vi "Configure Slider_Steering.vi"(8 "error in (no error)":errorcluster, 9 "NIVS.System Definition Root":refnum<k24>, 10 "VI Reference":refnum<vi>, 11 "Slide Parameters In":T1) -> (0 "error out":errorcluster, 3 "Slide Parameters Out":T1)   [LabVIEW 2013]
doc: "Use this template to create a dialog box with event handling."
uses:
  NationalInstruments.VeriStand.SystemStorage
  Support/Slide Parameters.ctl
  Support/PWM Object Parameters.ctl
  <vilib>/NI Veristand/UI Controls/Single Node Browser/NI_VS UI Single Node Browser.lvlib
  NationalInstruments.VeriStand.SystemStorageUI
panel:
  in  "Make Current Values Default":bool
  in  "Min Rail":dbl=0.1 min=0.0 max=1.0 step=0.0001
  in  "Max Rail":dbl=0.9 min=0.0 max=1.0 step=0.0001
  in  "BG color":u32(colorbox)=1245174
  in  "RIO?":bool caption="Hardware type"
  in  "Control Label":string
  out "PWM Config Tab":enum32{"DAQ", "RIO"}(tab)=enum."RIO"
  in  "OK":bool
  in  "Cancel":bool
  in  "Selected Channel":refnum<k24>(container)
  # "PWM Duty Cycle"
  # "LEFT"
  # "RIGHT"
  # "DAQ\nPWM\nRatio"
  # "FPGA\nPWM\n%"
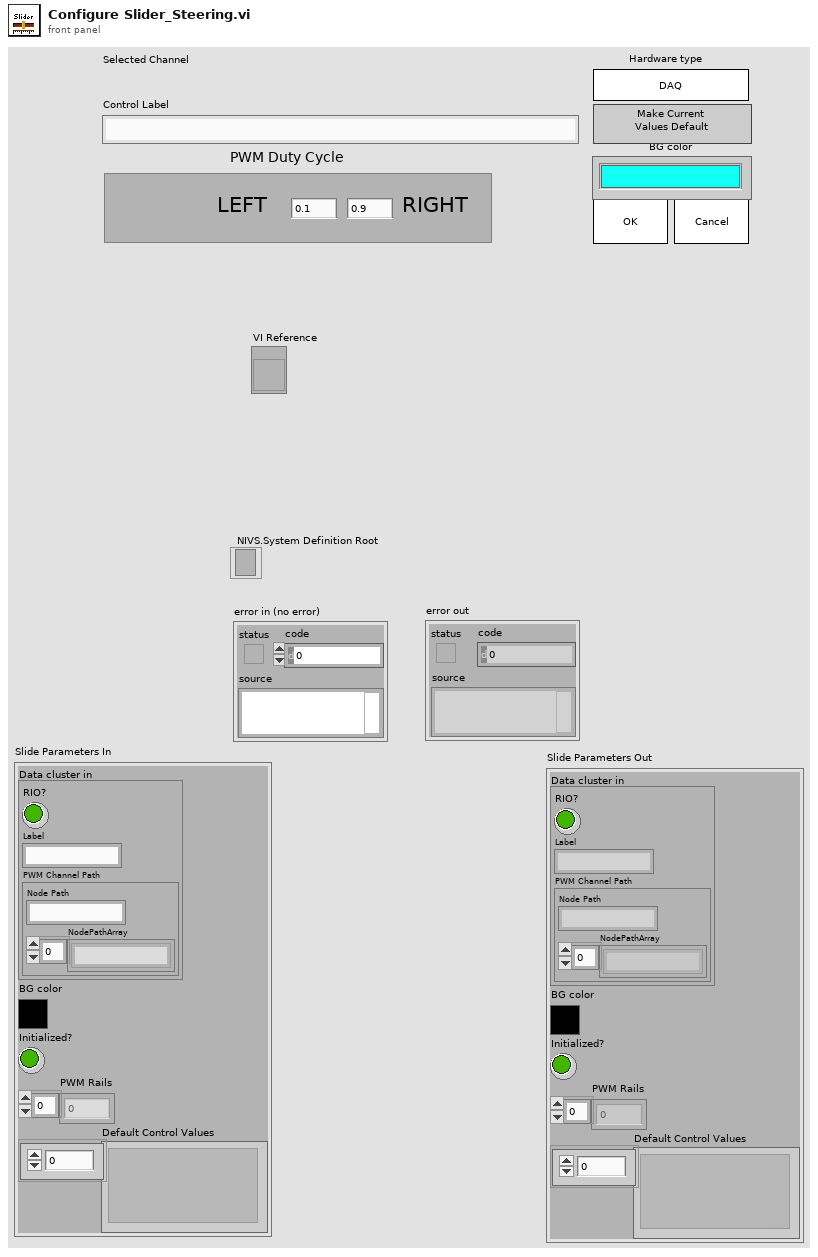
[diagram p1: front panel]
types:
  T1 = typedef "Slide Parameters.ctl" = cluster{"Data cluster in":T2, "BG color":u32, "Initialized?":bool, "PWM Rails":dbl[], "Default Control Values":variant[]}
  T2 = typedef "PWM Object Parameters.ctl" = cluster{"RIO?":bool, "Label":string, "PWM Channel Path":cluster{"NodePathArray":string[], "Node Path":string}}
  T3 = typedef "NI_VS UI Single Node Browser.lvlib/Callback Type.ctl" = cluster{"Net Callbacks":refnum<k27>[], "Event":refnum<user-event>}
  T4 = typedef "NI_VS UI Single Node Browser.lvlib/Node Ref.ctl" = refnum<k24>
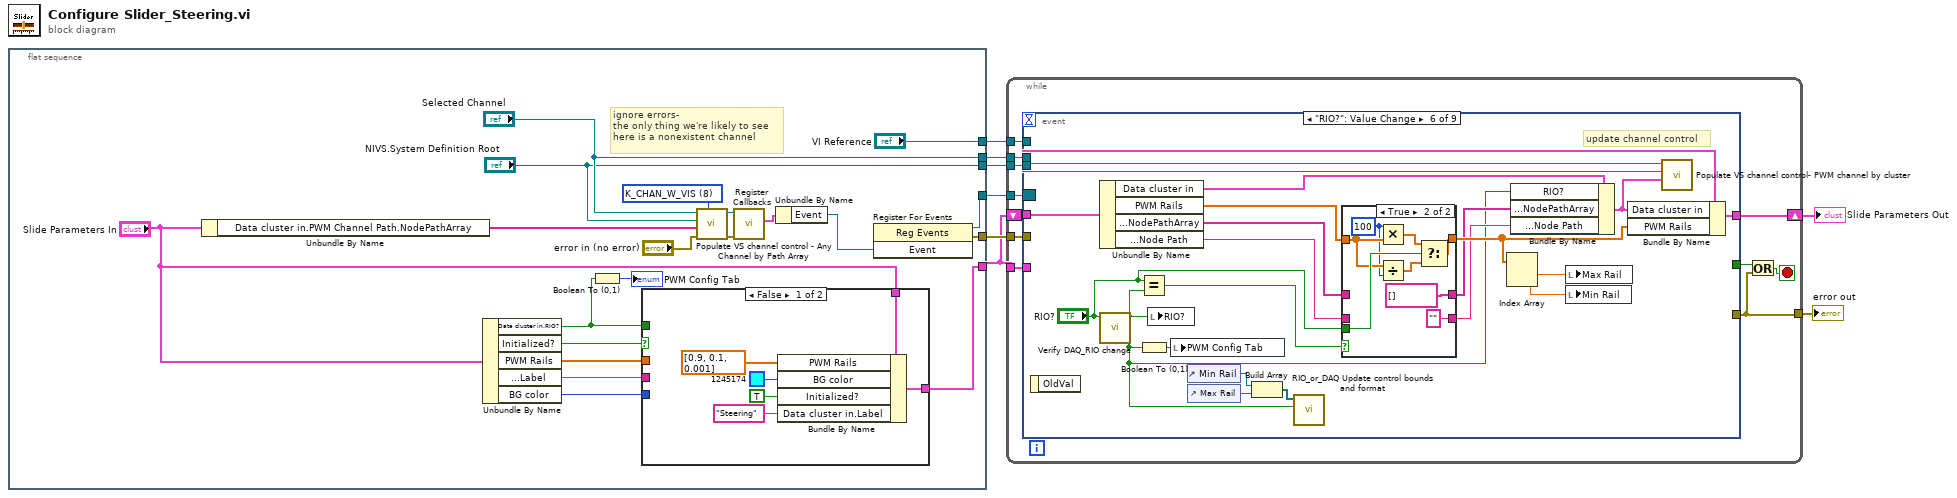
[diagram p0: block diagram]
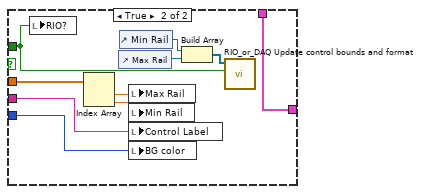
[diagram p2: hidden frame]
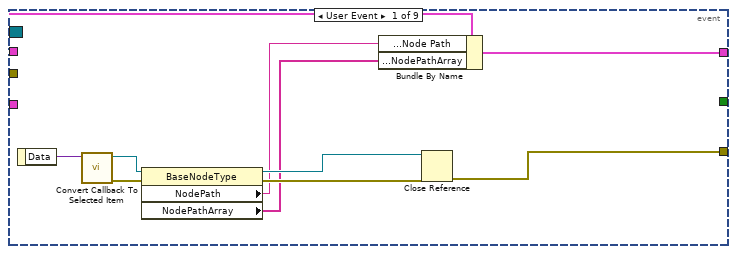
[diagram p3: hidden frame]
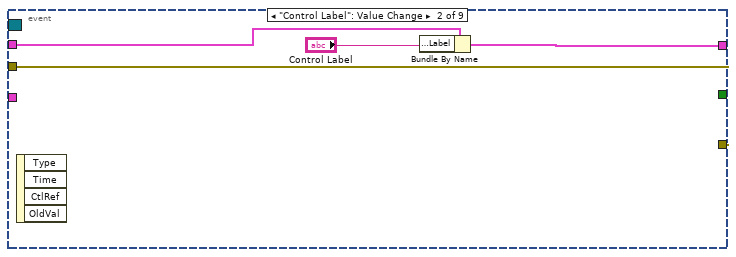
[diagram p4: hidden frame]
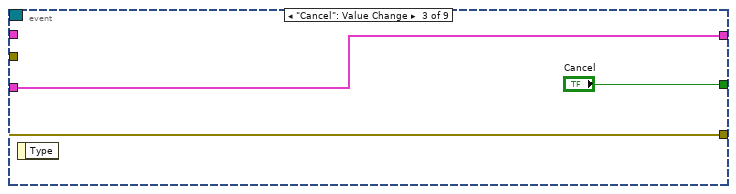
[diagram p5: hidden frame]
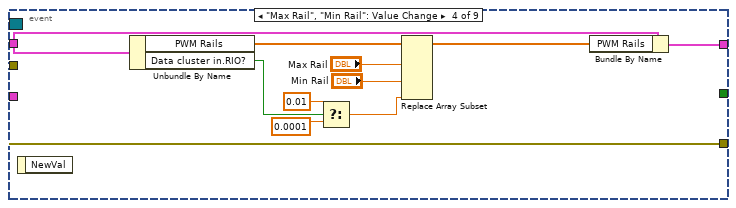
[diagram p6: hidden frame]
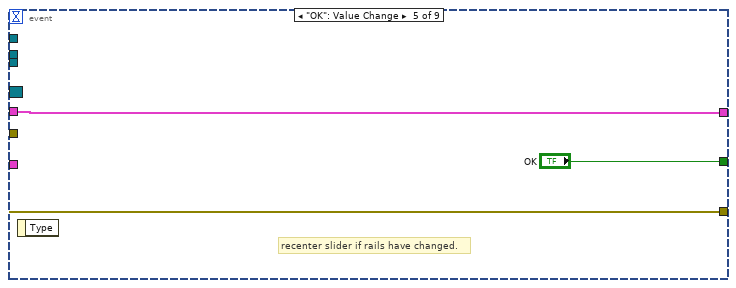
[diagram p7: hidden frame]
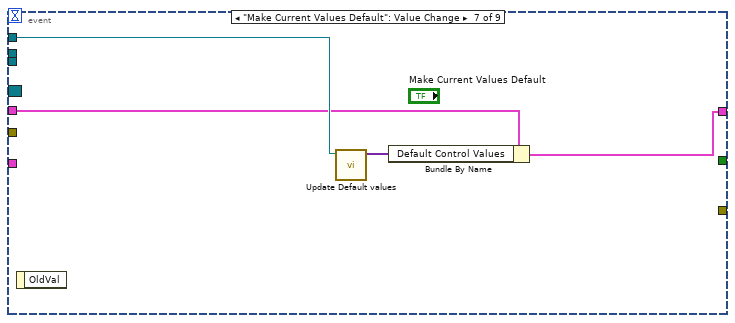
[diagram p9: hidden frame]
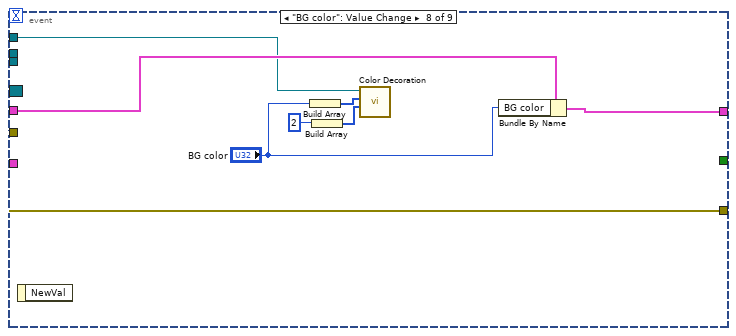
[diagram p10: hidden frame]
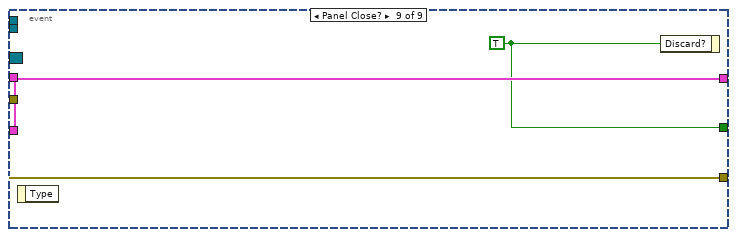
[diagram p11: hidden frame]
diagram:
  n1 = flat-sequence {
    tunnel: ["Selected Channel"] -> w7
    tunnel: ["NIVS.System Definition Root"] -> w6
    tunnel: [w13] -> w5
    tunnel: [w19] -> w4
    tunnel: ["VI Reference"] -> w3
    tunnel: [w12] -> w2
    frame #0 {
      w26 = u8 8 items=["K_CHAN_R", "K_CHAN_W", "K_CHAN_RW", "K_CHAN_VOLT", "K_CHAN_FAULT", "K_ALL", "K_CUSTOM", "K_CHAN_R_VIS", "K_CHAN_W_VIS", "K_CHAN_RW_VIS", "K_CHAN_VOLT_VIS", "K_CHAN_FAULT_VIS"] ("DisplayFilter")
      # "ignore errors-\nthe only thing we're likely to see\nhere is a nonexistent channel"
      n2 = Unbundle By Name("Slide Parameters In") -> ("Data cluster in.PWM Channel Path.NodePathArray"=w9:string[])
      n3 = Unbundle By Name("Slide Parameters In") -> ("Data cluster in.RIO?"=w10:bool, "Initialized?"=w20:bool, "PWM Rails"=w23:dbl[], "Data cluster in.Label"=w22:string, "BG color"=w21:u32)
      n4 = Boolean To (0,1)(Boolean=w10) -> (0, 1=→"PWM Config Tab":i16)
      n5 = case shown="False" w20 {
        tunnel: w23 -> [_ w43]
        tunnel: w22 -> [_ w42]
        tunnel: w21 -> [_ w41]
        tunnel: "Slide Parameters In" -> [w34 w40]
        tunnel: [w33 w40] -> w19
        tunnel: w10 -> [_ w37]
        frame False {
          n6 = Bundle By Name(cluster=w34, "PWM Rails"=dbl[] [0.9, 0.1, 0.001] ("RIO PWM Settings"), "BG color"=u32 1245174, "Initialized?"=TRUE ("New?"), "Data cluster in.Label"="Steering" ("Label")) -> (w33:T1)
        }
        frame True {
          n7 = local write "RIO?"(w37) -> ()
          n8 = Index Array(array=w43) -> (element #1=w44:dbl, element #2=w39:dbl)  [unwired: 2 in]
          n9 = control-ref of="Max Rail"() -> (w35:refnum<vi>)
          n10 = control-ref of="Min Rail"() -> (w36:refnum<vi>)
          n11 = local write "Max Rail"(w44) -> ()
          n12 = local write "Min Rail"(w39) -> ()
          n13 = local write "Control Label"(w42) -> ()
          n14 = local write "BG color"(w41) -> ()
          n15 = Build Array(w36, w35) -> (w38:refnum<vi>[])
          n16 = call "RIO_or_DAQ Update control bounds and format.vi"("RIO? in"=w37, "Control References in"=w38) -> ()  [unwired: 10 in]
        }
      }
      n17 = call "Populate VS channel control - Any Channel by Path Array.vi"("DisplayFilter"=w26, "error in (no error)"="error in (no error)", "Path Array In"=w9, "NIVS.System Definition Root"="NIVS.System Definition Root", ".NET Refnum in"="Selected Channel") -> ("error out"=w14:errorcluster, ".NET Refnum out"=w15:refnum<k24>)  [unwired: 5 in]
      n18 = call <vilib>:"Register Callbacks.vi"("error in (no error)"=w14, "Single Node Browser"=w15) -> ("Callbacks"=w17:T3)  [unwired: 7 in, 2 out]
      n19 = Unbundle By Name(w17) -> ("Event"=w16:refnum<user-event>)
      n20 = register-events(w16) -> (reference out=w12:refnum<event-registration>, error out=w13:errorcluster)  [unwired: 2 in]
    }
  }
  n21 = while {
    tunnel: [w45] -> w8
    shift-right: [w52] -> w1
    shift-left: w4 -> [w54]
    tunnel: w4 -> [w53]
    tunnel: w7 -> [w50]
    tunnel: w6 -> [w49]
    tunnel: w5 -> [w48]
    tunnel: w3 -> [w47]
    tunnel: w2 -> [w46]
    stop <- w51 stop-if-true
    n22 = event shown="[5] \"RIO?\": Value Change" {
      selector: w46 -> [_ _ _ _ _ _ _ _ _]
      dyn-events: _ -> [_ _ _ _ _ _ _ _ _]
      timeout: _ -> [_ _ _ _ _ _ _ _ _]
      tunnel: [_ _ "Cancel" _ "OK" _ _ _ w132] -> w55
      tunnel: [w57 w66 w70 w83 w85 _ _ w128 w131] -> w45
      tunnel: w54 -> [w58 w68 _ w81 w84 w104 w120 w129 _]
      tunnel: w53 -> [_ _ w71 _ _ _ _ _ w133]
      tunnel: [w56 w69 w71 w82 w84 w105 w119 w130 w133] -> w52
      tunnel: w50 -> [_ _ _ _ _ w107 _ _ _]
      tunnel: w49 -> [_ _ _ _ _ w106 _ _ _]
      tunnel: w48 -> [_ w66 w70 w83 w85 _ _ w128 w131]
      tunnel: w47 -> [_ _ _ _ _ _ w121 w125 _]
      event User Event {
        n23 = event-data() -> ("Data"=w59:variant)  [unwired: 1 in]
        n24 = call <vilib>:"Convert Callback To Selected Item.vi"("Data"=w59) -> ("error out"=w62:errorcluster, "Selected Item"=w65:T4)  [unwired: 9 in]
        n25 = property class="BaseNodeType"(reference=w65, error in=w62) -> (reference out=w64:T4, error out=w63:errorcluster, "NodePath"=w61:string, "NodePathArray"=w60:string[])
        n26 = Bundle By Name(cluster=w58, "Data cluster in.PWM Channel Path.Node Path"=w61, "Data cluster in.PWM Channel Path.NodePathArray"=w60) -> (w56:T1)
        n27 = Close Reference(reference=w64, error in (no error)=w63) -> (error out=w57:errorcluster)
      }
      event "Control Label": Value Change {
        n28 = event-data() -> ()  [unwired: 1 in, 4 out]
        n29 = Bundle By Name(cluster=w68, "Data cluster in.Label"="Control Label") -> (w69:T1)
      }
      event "Cancel": Value Change {
        n30 = event-data() -> ()  [unwired: 1 in, 1 out]
      }
      event "Max Rail", "Min Rail": Value Change {
        n31 = event-data() -> ()  [unwired: 1 in, 1 out]
        n32 = Unbundle By Name(w81) -> ("PWM Rails"=w78:dbl[], "Data cluster in.RIO?"=w74:bool)
        n33 = Select(t=0.01 ("element"), s=w74, f=0.0001 ("element")) -> (s? t:f=w75:dbl)
        n34 = Replace Array Subset(array=w78, new element #1="Max Rail", new element #2="Min Rail", new element #3=w75) -> (w77:dbl[])  [unwired: 3 in]
        n35 = Bundle By Name(cluster=w81, "PWM Rails"=w77) -> (w82:T1)
      }
      event "OK": Value Change {
        # "recenter slider if rails have changed."
        n36 = event-data() -> ()  [unwired: 1 in, 1 out]
      }
      event "RIO?": Value Change {
        # "update channel control"
        n37 = event-data() -> ()  [unwired: 1 in, 1 out]
        n38 = Unbundle By Name(w104) -> ("Data cluster in"=w103:T2, "PWM Rails"=w100:dbl[], "Data cluster in.PWM Channel Path.NodePathArray"=w99:string[], "Data cluster in.PWM Channel Path.Node Path"=w98:string)
        n39 = call "Verify DAQ_RIO change.vi"("RIO? in"="RIO?") -> ("RIO? out"=w87:bool)  [unwired: 10 in]
        n40 = Equal?(x="RIO?", y=w87) -> (x = y?=w97:bool)
        n41 = Boolean To (0,1)(Boolean=w87) -> (0, 1=w101:i16)
        n42 = local write "RIO?"(w87) -> ()
        n43 = local write "PWM Config Tab"(w101) -> ()
        n44 = control-ref of="Min Rail"() -> (w89:refnum<vi>)
        n45 = control-ref of="Max Rail"() -> (w88:refnum<vi>)
        n46 = Build Array(w89, w88) -> (w90:refnum<vi>[])
        n47 = call "RIO_or_DAQ Update control bounds and format.vi"("RIO? in"=w87, "Control References in"=w90) -> ()  [unwired: 10 in]
        n48 = case shown="True" w97 {
          tunnel: w100 -> [w110 w113]
          tunnel: "RIO?" -> [_ w117]
          tunnel: [w110 w116] -> w95
          tunnel: w99 -> [w109 _]
          tunnel: [w109 string[] [] ("NodePathArray")] -> w92
          tunnel: w98 -> [w108 _]
          tunnel: [w108 "" ("Node Path")] -> w91
          frame False {
          }
          frame True {
            w112 = 100
            n49 = Multiply(x=w112, y=w113) -> (x*y=w118:dbl[])
            n50 = Divide(x=w113, y=w112) -> (x/y=w115:dbl[])
            n51 = Select(t=w118, s=w117, f=w115) -> (s? t:f=w116:dbl[])
          }
        }
        n52 = Index Array(array=w95) -> (element #1=w94:dbl, element #2=w93:dbl)  [unwired: 2 in]
        n53 = Bundle By Name(cluster=w103, "RIO?"=w87, "PWM Channel Path.NodePathArray"=w92, "PWM Channel Path.Node Path"=w91) -> (w102:T2)
        n54 = local write "Max Rail"(w94) -> ()
        n55 = local write "Min Rail"(w93) -> ()
        n56 = Bundle By Name(cluster=w104, "Data cluster in"=w102, "PWM Rails"=w95) -> (w105:T1)
        n57 = call "Populate VS channel control- PWM channel by cluster.vi"("Data cluster in"=w102, "NIVS.System Definition Root"=w106, ".NET Refnum in"=w107) -> ()  [unwired: 7 in, 2 out]
      }
      event "Make Current Values Default": Value Change {
        n58 = event-data() -> ()  [unwired: 1 in, 1 out]
        n59 = call "Update Default values.vi"("VI in"=w121) -> ("Default Values out"=w122:variant[])  [unwired: 10 in]
        n60 = Bundle By Name(cluster=w120, "Default Control Values"=w122) -> (w119:T1)
      }
      event "BG color": Value Change {
        n61 = event-data() -> ()  [unwired: 1 in, 1 out]
        n62 = Build Array("BG color") -> (w127:u32[])
        n63 = Build Array(u32 2 ("BG color out")) -> (w124:u32[])
        n64 = call "Color Decoration.vi"("VI reference"=w125, "Color Array"=w127, "Index Array"=w124) -> ()  [unwired: 7 in, 1 out]
        n65 = Bundle By Name(cluster=w129, "BG color"="BG color") -> (w130:T1)
      }
      event Panel Close? {
        w132 = TRUE ("Cancel")
        n66 = event-data() -> ()  [unwired: 1 in, 1 out]
        n67 = event-data("Discard?"=w132) -> ()  [unwired: 1 in, 1 out]
      }
    }
    n68 = Or(x=w55, y=w45) -> (x .or. y?=w51:bool)
  }
  "error out" <- w8
  "Slide Parameters Out" <- w1
